vi "Pos ctrl window-Initialise control values.vi"(11 "Pos ctrl window refs":T1) -> (0 "error out":errorcluster)   [LabVIEW 2020]
uses:
  Typedefs/Pos Ctrl window refs cluster.ctl
  <userlib>/My Palettes.lib/Custom Controls/Directional Arrow Buttons/Arrow button-North.ctl
  Peripherals Control/XYZ Stage/Typedefs/XYZ stage states.ctl
  Globals/Pos ctrl window globals.vi
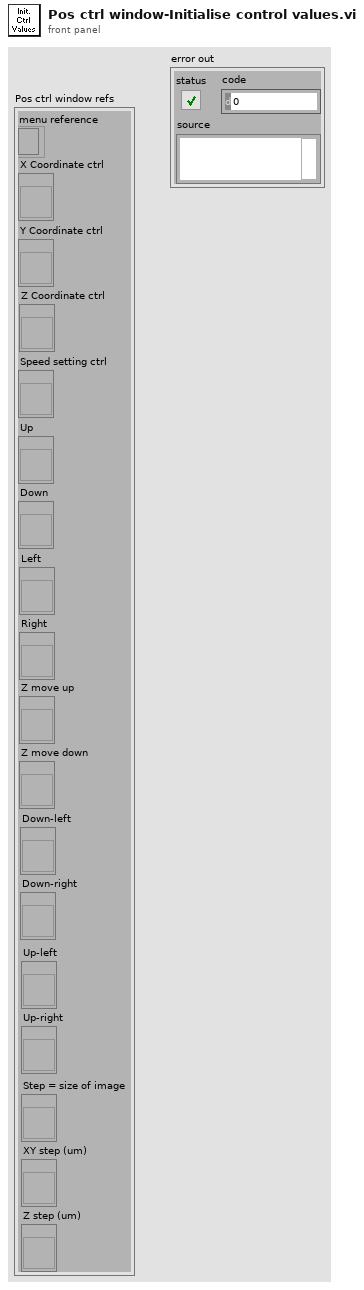
[diagram p1: front panel]
types:
  T1 = typedef "Pos Ctrl window refs cluster.ctl" = cluster{"menu reference":refnum<k9>, "X Coordinate ctrl":refnum<vi>, "Y Coordinate ctrl":refnum<vi>, "Z Coordinate ctrl":refnum<vi>, "Speed setting ctrl":refnum<vi>, "Up":refnum<vi>, "Down":refnum<vi>, "Left":refnum<vi>, "Right":refnum<vi>, "Z move up":refnum<vi>, "Z move down":refnum<vi>, "Down-left":refnum<vi>, "Down-right":refnum<vi>, "Up-left":refnum<vi>, "Up-right":refnum<vi>, "Step = size of image":refnum<vi>, "XY step (um)":refnum<vi>, "Z step (um)":refnum<vi>}
  T2 = typedef "XYZ stage states.ctl" = enum16{"Dequeue", "Initialize", "Read Position", "Read Speed Setting", "Move", "Set Max Speed", "Reset Axis", "Stop all movement"}
  T3 = enum8{"Enabled", "Disabled", "Disabled and Grayed Out"}
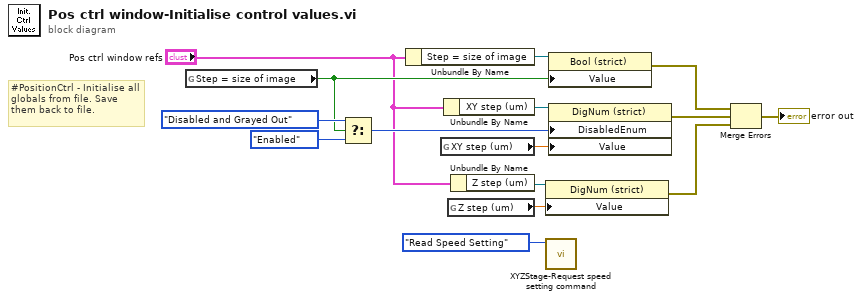
[diagram p0: block diagram]
diagram:
  # "#PositionCtrl - Initialise all globals from file. Save them back to file."
  n1 = global read "Pos ctrl window globals.vi" "Step = size of image"() -> (w11:bool)
  n2 = Select(t=T3."Disabled and Grayed Out" ("Disabled"), s=w11, f=T3."Enabled" ("Disabled")) -> (s? t:f=w14:T3)
  n3 = Unbundle By Name("Pos ctrl window refs") -> ("Step = size of image"=w9:refnum<vi>)
  n4 = global read "Pos ctrl window globals.vi" "XY step (um)"() -> (w12:sgl)
  n5 = Unbundle By Name("Pos ctrl window refs") -> ("XY step (um)"=w8:refnum<vi>)
  n6 = global read "Pos ctrl window globals.vi" "Z step (um)"() -> (w10:sgl)
  n7 = Unbundle By Name("Pos ctrl window refs") -> ("Z step (um)"=w7:refnum<vi>)
  n8 = property on="Property Node" class="DigNum (strict)"(reference=w7, "Value"=w10) -> (error out=w4:errorcluster)  [unwired: 1 in, 1 out]
  n9 = call "XYZStage-Request speed setting command.vi"("Which speed setting command?"=XYZ_stage_states."Read Speed Setting" ("Command")) -> ()  [unwired: 10 in, 1 out]
  n10 = property on="Property Node" class="Bool (strict)"(reference=w9, "Value"=w11) -> (error out=w6:errorcluster)  [unwired: 1 in, 1 out]
  n11 = property on="Property Node" class="DigNum (strict)"(reference=w8, "DisabledEnum"=w14, "Value"=w12) -> (error out=w5:errorcluster)  [unwired: 1 in, 1 out]
  n12 = Merge Errors(w6, w5, w4) -> (→"error out":errorcluster)
